vi "Query List Step Duration Time.vi"(8 "error in (no error)":errorcluster {"code" format="%.0x"}, 9 "StepIndex":i32 format="%.0g", 11 "instrument handle":refnum<k15>) -> (0 "error out":errorcluster {"code" format="%.0x"}, 2 "Val":dbl, 3 "instrument handle out":refnum<k15>)   [LabVIEW 2009, in "Keysight XSAn.lvlib"]
doc: "Query the length of time the step will play.\n\nSupported Models: M8920A, M9420A, M9421A."
uses:
  <instrlib>/Keysight XSAn/Keysight XSAn.lvlib
  AgXSAn.dll
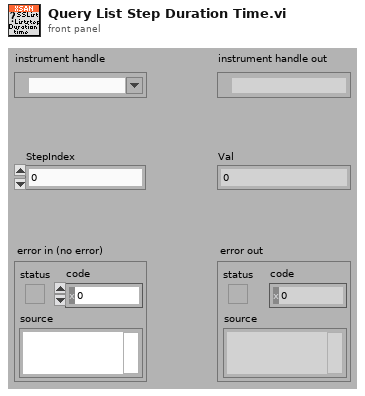
[diagram p1: front panel]
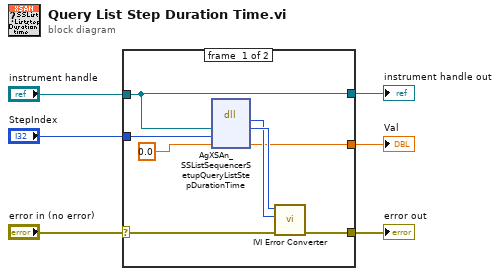
[diagram p0: block diagram]
diagram:
  n1 = case shown="No Error" "error in (no error)" {
    selector: "error in (no error)" -> [w12 w16]
    tunnel: [w11 w16] -> w6
    tunnel: "instrument handle" -> [w7 w15]
    tunnel: "StepIndex" -> [w10 _]
    tunnel: [w8 _] -> w2
    tunnel: [w7 w15] -> w1
    frame #0 {
      n2 = dll-call lib="AgXSAn**.dll" fn="AgXSAn_SSListSequencerSetupQueryListStepDurationTime"("Vi"=w7, "StepIndex"=w10, "Val"=0.0) -> (w13:i32, "Vi"=w14:u32, "Val"=w8:dbl)  [unwired: 4 in, 2 out]
      n3 = call <instrlib>:"IVI Error Converter.vi"("error in (no error)"=w12, "IVI error code (0)"=w13, "instrument handle"=w14) -> ("error out"=w11:errorcluster)  [unwired: 7 in, 1 out]
    }
    frame #1 {
    }
  }
  "error out" <- w6
  "instrument handle out" <- w1
  "Val" <- w2
